vi "testfit.vi"() -> ()   [LabVIEW 2012]
panel:
  out "X":dbl[](array[numeric])
  out "coef":dbl[](array[numeric])
  in  "Tan":dbl[](array[numeric])
  in  "DO":dbl[](array[numeric])
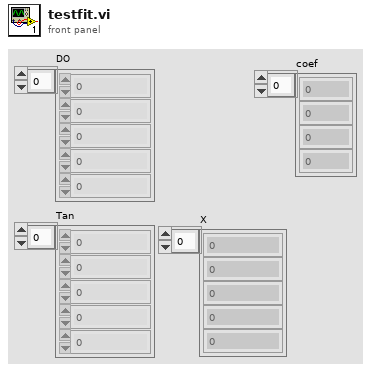
[diagram p1: front panel]
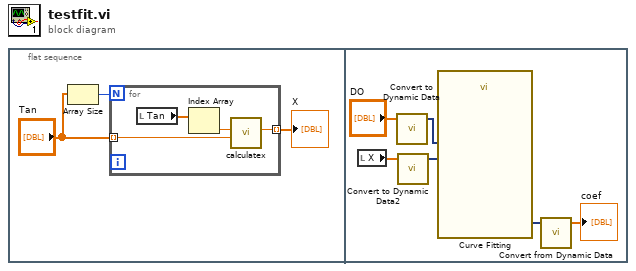
[diagram p0: block diagram]
diagram:
  n1 = flat-sequence {
    frame #0 {
      n2 = Array Size(array="Tan") -> (size(s)=w3:i32)
      n3 = for {
        N: w3 -> [_]
        tunnel: "Tan" -> [w7] mode=indexing
        tunnel: [w6] -> w1 mode=indexing
        n4 = local read "Tan"() -> (w5:dbl[])
        n5 = Index Array(array=w5) -> (element=w4:dbl)  [unwired: 1 in]
        n6 = call "calculatex.vi"("T"=w7, "T0"=w4) -> ("X"=w6:dbl)  [unwired: 9 in]
      }
      "X" <- w1
    }
    frame #1 {
      n7 = local read "X"() -> (w9:dbl[])
      n8 = call "Convert to Dynamic Data"("Array"="DO") -> ("Dynamic Data Type"=w12:dynamicdata)  [unwired: 3 in]
      n9 = call "Convert to Dynamic Data2"("Array"=w9) -> ("Dynamic Data Type"=w8:dynamicdata)  [unwired: 3 in]
      n10 = call "Curve Fitting"("Locations"=w8, "Signals"=w12) -> ("polynomial coefficients"=w11:dynamicdata)  [unwired: 5 in, 4 out]
      n11 = call "Convert from Dynamic Data"("Dynamic Data Type"=w11) -> ("Array"=→"coef":dbl[])  [unwired: 3 in]
    }
  }
